vi "Initialize_Queues.vi"(8 "Status/Errors in":refnum<vi>) -> (0 "Status/Errors out":refnum<vi>, 4 "Queues":T1)   [LabVIEW 2013]
uses:
  Controls/Queues.ctl
  Controls/One_Second.ctl
  Controls/GPS_Timestamp.ctl
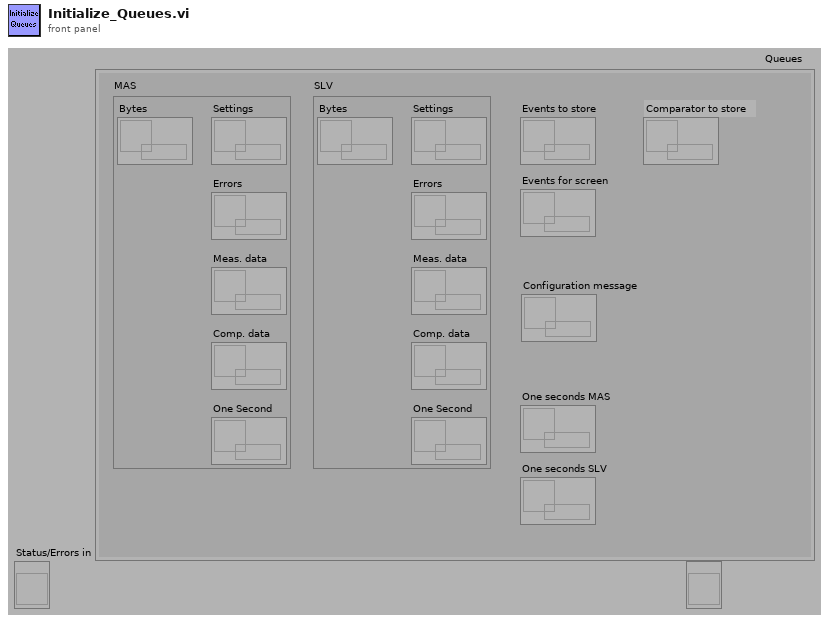
[diagram p1: front panel]
types:
  T1 = typedef "Queues.ctl" = cluster{"MAS":cluster{"Bytes":refnum<queue>, "Settings":refnum<queue>, "Errors":refnum<queue>, "Meas. data":refnum<queue>, "One Second":refnum<queue>, "Comp. data":refnum<queue>}, "SLV":cluster{"Bytes":refnum<queue>, "Settings":refnum<queue>, "Errors":refnum<queue>, "Meas. data":refnum<queue>, "One Second":refnum<queue>, "Comp. data":refnum<queue>}, "Events to store":refnum<queue>, "Events for screen":refnum<queue>, "One seconds MAS":refnum<queue>, "One seconds SLV":refnum<queue>, "Configuration message":refnum<queue>, "Comparator to store":refnum<queue>}
  T2 = typedef "One_Second.ctl" = cluster{"GPS timestamp":T3, "CTP":u32, "Quantization error":u32, "Ch1 High":u16, "Ch1 Low":u16, "Ch2 High":u16, "Ch2 Low":u16, "Event rate":u16, "# Satellites":u8, "Satellite 1":u8, "Satellite 2":u8, "Satellite 3":u8, "Satellite 4":u8, "Satellite 5":u8, "Satellite 6":u8, "Signal level 1":sgl, "Signal level 2":sgl, "Signal level 3":sgl, "Signal level 4":sgl, "Signal level 5":sgl, "Signal level 6":sgl, "Satellite 7":u8, "Satellite 8":u8, "Satellite 9":u8, "Satellite 10":u8, "Satellite 11":u8, "Satellite 12":u8, "Signal level 7":sgl, "Signal level 8":sgl, "Signal level 9":sgl, "Signal level 10":sgl, "Signal level 11":sgl, "Signal level 12":sgl}
  T3 = typedef "GPS_Timestamp.ctl" = cluster{"Seconds":u8, "Minutes":u8, "Hours":u8, "Day":u8, "Month":u8, "Year":u16}
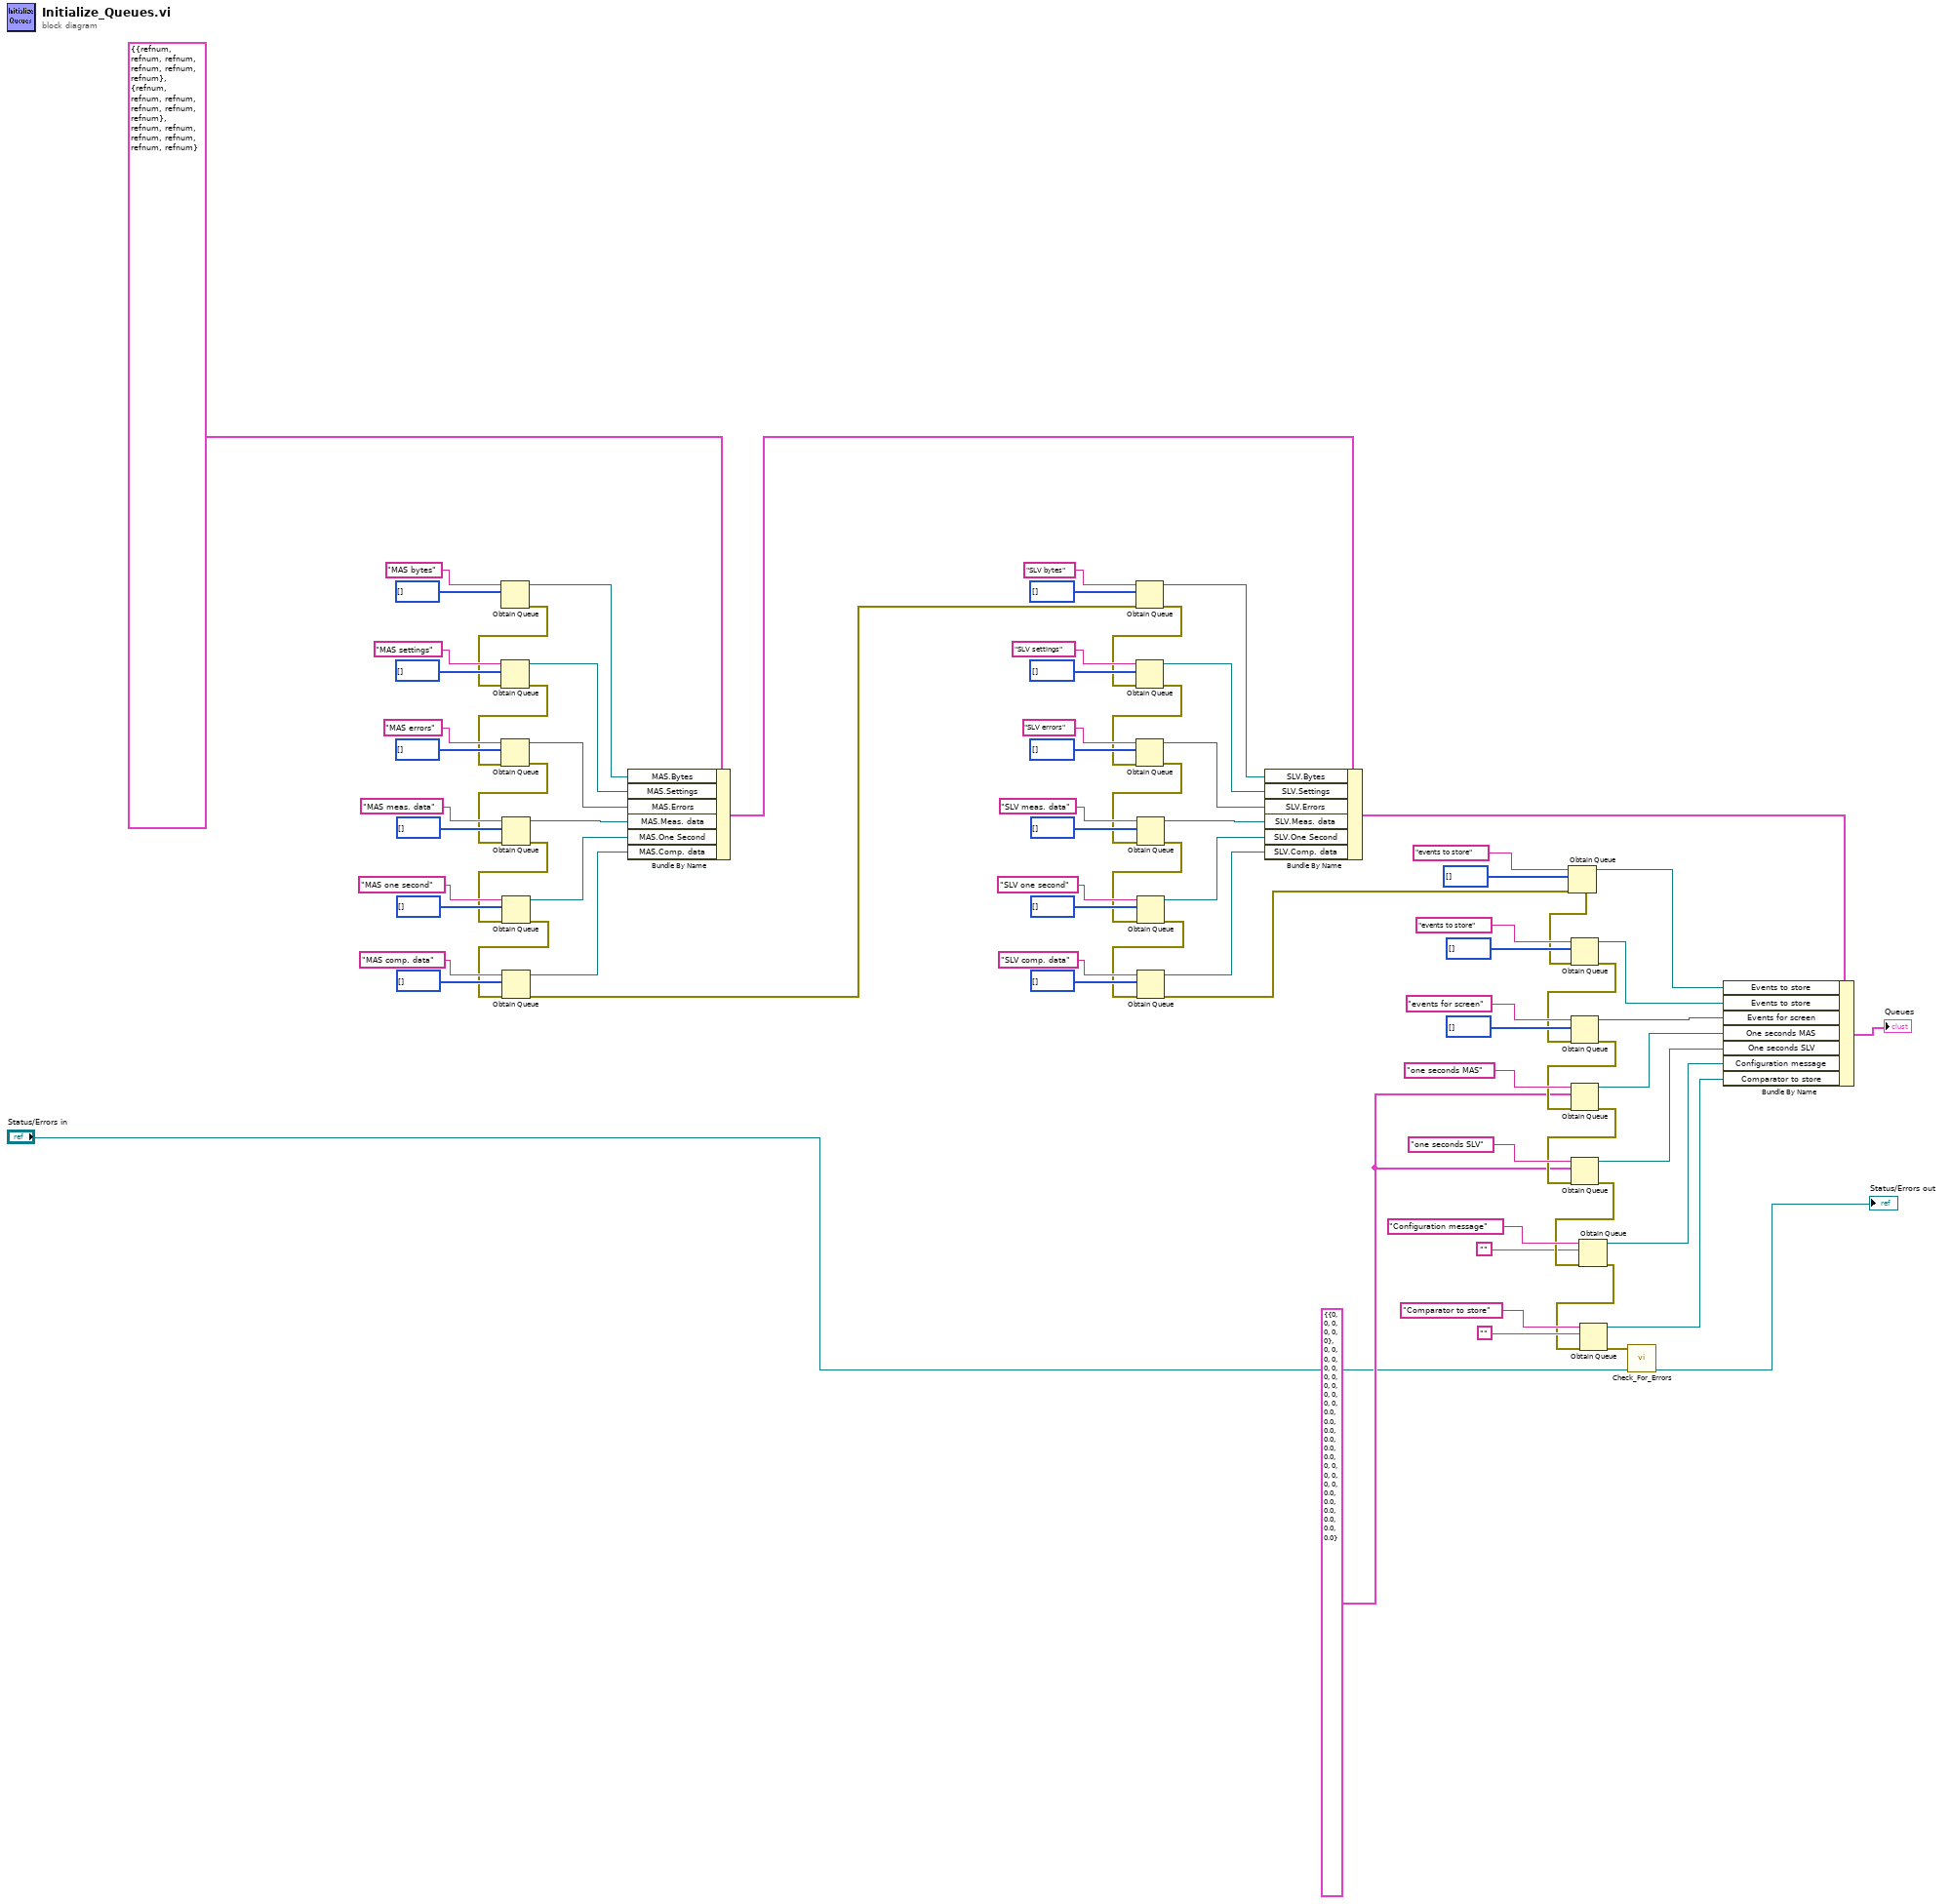
[diagram p0: block diagram]
diagram:
  w17 = T2 {"GPS timestamp"={"Seconds"=0, "Minutes"=0, "Hours"=0, "Day"=0, "Month"=0, "Year"=0}, "CTP"=0, "Quantization error"=0, "Ch1 High"=0, "Ch1 Low"=0, "Ch2 High"=0, "Ch2 Low"=0, "Event rate"=0, "# Satellites"=0, "Satellite 1"=0, "Satellite 2"=0, "Satellite 3"=0, "Satellite 4"=0, "Satellite 5"=0, "Satellite 6"=0, "Signal level 1"=0.0, "Signal level 2"=0.0, "Signal level 3"=0.0, "Signal level 4"=0.0, "Signal level 5"=0.0, "Signal level 6"=0.0, "Satellite 7"=0, "Satellite 8"=0, "Satellite 9"=0, "Satellite 10"=0, "Satellite 11"=0, "Satellite 12"=0, "Signal level 7"=0.0, "Signal level 8"=0.0, "Signal level 9"=0.0, "Signal level 10"=0.0, "Signal level 11"=0.0, "Signal level 12"=0.0} ("One second")
  n1 = Obtain Queue(name (unnamed)="MAS bytes", element data type=u8[] []) -> (queue out=w79:refnum<queue>, error out=w66:errorcluster)  [unwired: 3 in, 1 out]
  n2 = Obtain Queue(name (unnamed)="MAS settings", element data type=u8[] [], error in (no error)=w66) -> (queue out=w70:refnum<queue>, error out=w65:errorcluster)  [unwired: 2 in, 1 out]
  n3 = Obtain Queue(name (unnamed)="MAS errors", element data type=u8[] [], error in (no error)=w65) -> (queue out=w69:refnum<queue>, error out=w64:errorcluster)  [unwired: 2 in, 1 out]
  n4 = Obtain Queue(name (unnamed)="MAS meas. data", element data type=u8[] [], error in (no error)=w64) -> (queue out=w68:refnum<queue>, error out=w63:errorcluster)  [unwired: 2 in, 1 out]
  n5 = Obtain Queue(name (unnamed)="MAS one second", element data type=u8[] [], error in (no error)=w63) -> (queue out=w67:refnum<queue>, error out=w51:errorcluster)  [unwired: 2 in, 1 out]
  n6 = Obtain Queue(name (unnamed)="MAS comp. data", element data type=u8[] [], error in (no error)=w51) -> (queue out=w50:refnum<queue>, error out=w26:errorcluster)  [unwired: 2 in, 1 out]
  n7 = Bundle By Name(cluster=T1 {"MAS"={"Bytes"=refnum, "Settings"=refnum, "Errors"=refnum, "Meas. data"=refnum, "One Second"=refnum, "Comp. data"=refnum}, "SLV"={"Bytes"=refnum, "Settings"=refnum, "Errors"=refnum, "Meas. data"=refnum, "One Second"=refnum, "Comp. data"=refnum}, "Events to store"=refnum, "Events for screen"=refnum, "One seconds MAS"=refnum, "One seconds SLV"=refnum, "Configuration message"=refnum, "Comparator to store"=refnum} ("Queues"), "MAS.Bytes"=w79, "MAS.Settings"=w70, "MAS.Errors"=w69, "MAS.Meas. data"=w68, "MAS.One Second"=w67, "MAS.Comp. data"=w50) -> (w25:T1)
  n8 = Obtain Queue(name (unnamed)="SLV bytes", element data type=u8[] [], error in (no error)=w26) -> (queue out=w47:refnum<queue>, error out=w34:errorcluster)  [unwired: 2 in, 1 out]
  n9 = Obtain Queue(name (unnamed)="SLV settings", element data type=u8[] [], error in (no error)=w34) -> (queue out=w38:refnum<queue>, error out=w33:errorcluster)  [unwired: 2 in, 1 out]
  n10 = Obtain Queue(name (unnamed)="SLV errors", element data type=u8[] [], error in (no error)=w33) -> (queue out=w37:refnum<queue>, error out=w32:errorcluster)  [unwired: 2 in, 1 out]
  n11 = Obtain Queue(name (unnamed)="SLV meas. data", element data type=u8[] [], error in (no error)=w32) -> (queue out=w36:refnum<queue>, error out=w31:errorcluster)  [unwired: 2 in, 1 out]
  n12 = Obtain Queue(name (unnamed)="SLV one second", element data type=u8[] [], error in (no error)=w31) -> (queue out=w35:refnum<queue>, error out=w28:errorcluster)  [unwired: 2 in, 1 out]
  n13 = Obtain Queue(name (unnamed)="SLV comp. data", element data type=u8[] [], error in (no error)=w28) -> (queue out=w27:refnum<queue>, error out=w13:errorcluster)  [unwired: 2 in, 1 out]
  n14 = Bundle By Name(cluster=w25, "SLV.Bytes"=w47, "SLV.Settings"=w38, "SLV.Errors"=w37, "SLV.Meas. data"=w36, "SLV.One Second"=w35, "SLV.Comp. data"=w27) -> (w24:T1)
  n15 = Obtain Queue(name (unnamed)="events to store", element data type=u8[] [], error in (no error)=w13) -> (queue out=w14:refnum<queue>, error out=w12:errorcluster)  [unwired: 2 in, 1 out]
  n16 = Obtain Queue(name (unnamed)="events to store", element data type=u8[] [], error in (no error)=w12) -> (queue out=w55:refnum<queue>, error out=w56:errorcluster)  [unwired: 2 in, 1 out]
  n17 = Obtain Queue(name (unnamed)="events for screen", element data type=u8[] [], error in (no error)=w56) -> (queue out=w54:refnum<queue>, error out=w20:errorcluster)  [unwired: 2 in, 1 out]
  n18 = Obtain Queue(name (unnamed)="one seconds MAS", element data type=w17, error in (no error)=w20) -> (queue out=w19:refnum<queue>, error out=w21:errorcluster)  [unwired: 2 in, 1 out]
  n19 = Obtain Queue(name (unnamed)="one seconds SLV", element data type=w17, error in (no error)=w21) -> (queue out=w18:refnum<queue>, error out=w10:errorcluster)  [unwired: 2 in, 1 out]
  n20 = Obtain Queue(name (unnamed)="Configuration message", element data type="", error in (no error)=w10) -> (queue out=w9:refnum<queue>, error out=w1:errorcluster)  [unwired: 2 in, 1 out]
  n21 = Obtain Queue(name (unnamed)="Comparator to store", element data type="", error in (no error)=w1) -> (queue out=w2:refnum<queue>, error out=w6:errorcluster)  [unwired: 2 in, 1 out]
  n22 = call "Check_For_Errors.vi"("Status/Errors in"="Status/Errors in", "error in"=w6) -> ("Status/Errors out"=→"Status/Errors out":refnum<vi>)  [unwired: 9 out]
  n23 = Bundle By Name(cluster=w24, "Events to store"=w14, "Events to store"=w55, "Events for screen"=w54, "One seconds MAS"=w19, "One seconds SLV"=w18, "Configuration message"=w9, "Comparator to store"=w2) -> (→"Queues":T1)
